vi "Disabled.vi"(7 "Robot Mode":T2, 10 "Match Info":T1={"Autonomous Elapsed Seconds"=0.0, "TeleOp Elapsed Seconds"=0.0, "Disabled Elapsed Seconds"=0.0, "Visited Autonomous"=FALSE, "Visited TeleOp"=FALSE, "Visited Disabled"=FALSE, "Autonomous Settings"={"Autonomous Style"=enum."Independent", "VI Refnum"=refnum}}, 11 "Call Context":T3) -> ()   [LabVIEW 2013]
doc: "This VI is called each time a disabled packet is received from the DS. It is often used to prepare for the next robot mode, to calibrate sensors, etc."
uses:
  <vilib>/Rock Robotics/WPI/DriverStation/WPI_DriverStationDerivedRobotMode.ctl
  <vilib>/Rock Robotics/WPI/DriverStation/WPI_DriverStationRobotMode2.ctl
  <vilib>/Rock Robotics/WPI/DriverStation/WPI_DriverStationMatch Info.ctl
  <vilib>/Rock Robotics/WPI/Solenoid/WPI_SolenoidValue.ctl
  Systems/Intake/Intake Global.vi
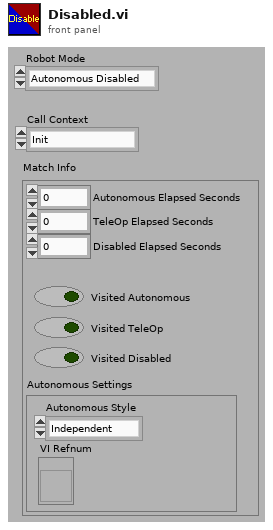
[diagram p1: front panel]
types:
  T1 = typedef "WPI_DriverStationMatch Info.ctl" = cluster{"Autonomous Elapsed Seconds":dbl, "TeleOp Elapsed Seconds":dbl, "Disabled Elapsed Seconds":dbl, "Visited Autonomous":bool, "Visited TeleOp":bool, "Visited Disabled":bool, "Autonomous Settings":cluster{"Autonomous Style":enum16{"Iterative", "Independent"}, "VI Refnum":refnum<vi>}}
  T2 = typedef "WPI_DriverStationRobotMode2.ctl" = enum16{"Autonomous Disabled", "Autonomous Enabled", "Teleop Disabled", "Teleop Enabled", "Timeout", "Finish", "Test Disabled", "Test Enabled"}
  T3 = typedef "WPI_DriverStationDerivedRobotMode.ctl" = enum16{"Init", "Execute", "Stop"}
  T4 = typedef "WPI_SolenoidValue.ctl" = enum16{"Off", "On", "Forward", "Reverse"}
  T5 = typedef "WPI_RelayValue.ctl" = enum16{"Off", "On", "Forward", "Reverse"}
  T6 = cluster{"Arm State":bool, "Gripper In":bool, "Gripper Out":bool, "Gripper Execution":T5, "Arm Execution":T4, "Middle MS":bool, "Middle Stop":bool}
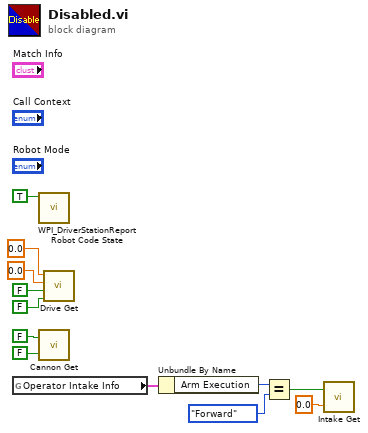
[diagram p0: block diagram]
diagram:
  n1 = global read "Intake Global.vi" "Operator Intake Info"() -> (w7:T6)
  n2 = call <vilib>:"WPI_DriverStationReport Robot Code State.vi"("Disabled"=TRUE ("Autonomous")) -> ()  [unwired: 10 in, 1 out]
  n3 = call "Cannon Get.vi"("Arm?"=FALSE ("Gripper  Out"), "Le Fire At Will?"=FALSE ("Gripper In")) -> ()  [unwired: 1 in]
  n4 = call "Drive Get.vi"("Show off spin"=FALSE, "Slow Drive"=FALSE, "Y - Axis"=0.0, "X - Axis"=0.0) -> ()  [unwired: 8 in]
  n5 = Unbundle By Name(w7) -> ("Arm Execution"=w6:T4)
  n6 = Equal?(x=w6, y=WPI_SolenoidValue."Forward" ("Arm Execution")) -> (x = y?=w4:bool)
  n7 = call "Intake Get.vi"("Gripper"=0.0, "Arm State"=w4) -> ()  [unwired: 1 in]
